vi "Build Async Parameters.vi"(8 "Error in":errorcluster, 11 "State Vars":T4 {"CompiledSettings"."Result Ch Data Refs" format="%.0x"; "CompiledSettings"."Parameter Block Data Refs"."Data Reference" format="%.0x"}) -> (0 "Error out":errorcluster, 2 "Async Parameters":T1, 3 "State Vars out":T4 {"CompiledSettings"."Result Ch Data Refs" format="%.0x"; "CompiledSettings"."Parameter Block Data Refs"."Data Reference" format="%.0x"})   [LabVIEW 2015, in "Waveform-Processing-Custom-Device Engine.lvlib"]
uses:
  Waveform-Processing-Custom-Device Engine.lvlib
  Types/Inline State Vars.ctl
  Types/Async FIFOs.ctl
  Shared/CompiledSettings.ctl
  <vilib>/NI Veristand/Custom Device API/Block Data Reference.ctl
  Built/Waveform-Processing-Custom-Device/Waveform-Processing-Custom-Device Engine Windows.llb/Data Reference.ctl
  <vilib>/NI Veristand/Custom Device API/Waveform Data Reference.ctl
  Types/Async Parameters.ctl
  <vilib>/NI VeriStand/Custom Device API/Custom Device API.lvlib
  Shared/Waveform-Processing-Custom-Device Shared.lvlib
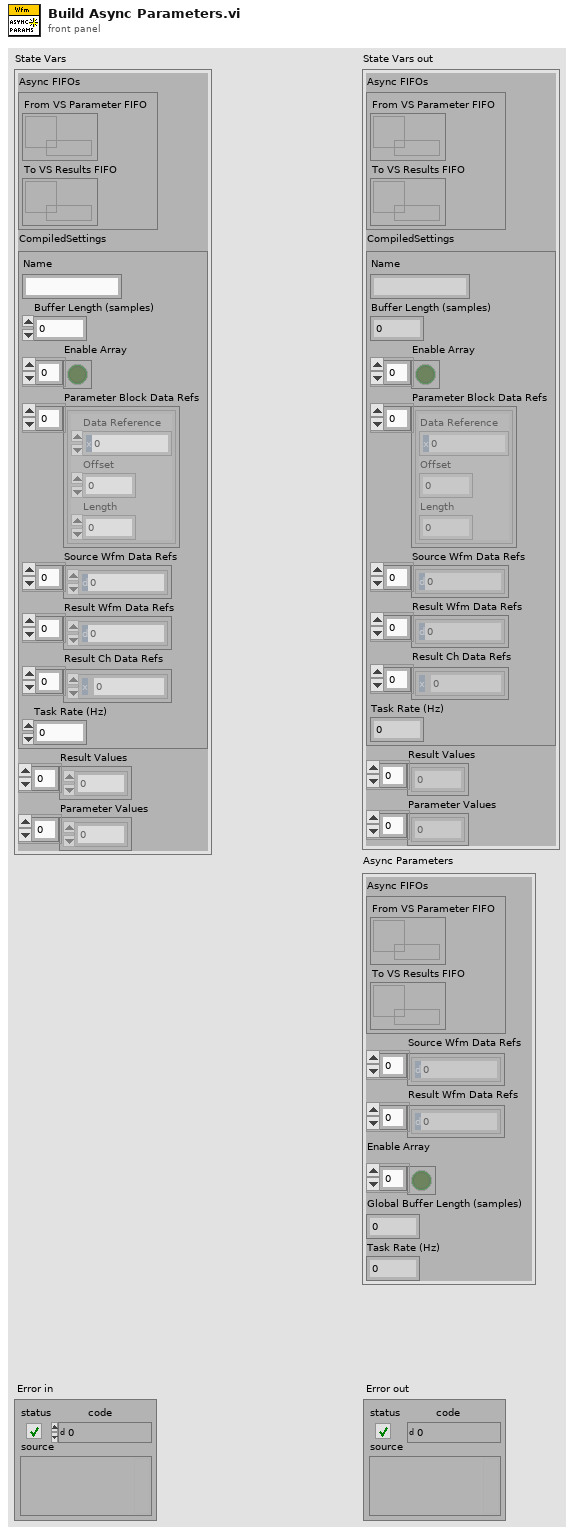
[diagram p1: front panel]
types:
  T1 = typedef "Waveform-Processing-Custom-Device Engine.lvlib/Async Parameters.ctl" = cluster{"Async FIFOs":T2, "Source Wfm Data Refs":T3[], "Result Wfm Data Refs":T3[], "Enable Array":bool[], "Global Buffer Length (samples)":dbl, "Task Rate (Hz)":dbl}
  T2 = typedef "Waveform-Processing-Custom-Device Engine.lvlib/Async FIFOs.ctl" = cluster{"From VS Parameter FIFO":refnum<k33>, "To VS Results FIFO":refnum<k33>}
  T3 = typedef "Custom Device API.lvlib/Waveform Data Reference.ctl" = i32
  T4 = typedef "Waveform-Processing-Custom-Device Engine.lvlib/Inline State Vars.ctl" = cluster{"Async FIFOs":T2, "CompiledSettings":T5, "Result Values":dbl[], "Parameter Values":dbl[]}
  T5 = typedef "Waveform-Processing-Custom-Device Shared.lvlib/CompiledSettings.ctl" = cluster{"Name":string, "Buffer Length (samples)":u32, "Enable Array":bool[], "Parameter Block Data Refs":T6[], "Source Wfm Data Refs":T3[], "Result Wfm Data Refs":T3[], "Result Ch Data Refs":T7[], "Task Rate (Hz)":dbl}
  T6 = typedef "Custom Device API.lvlib/Block Data Reference.ctl" = cluster{"Data Reference":T7, "Offset":u64, "Length":u64}
  T7 = typedef "Custom Device API.lvlib/Data Reference.ctl" = i32
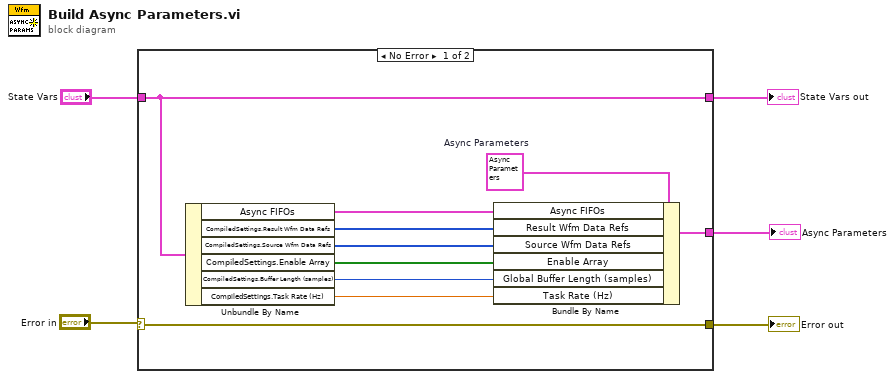
[diagram p0: block diagram]
diagram:
  n1 = case shown="No Error" "Error in" {
    selector: "Error in" -> [w11 w17]
    tunnel: [w11 w17] -> w4
    tunnel: "State Vars" -> [w12 w16]
    tunnel: [w12 w16] -> w2
    tunnel: [w13 _] -> w1
    frame No Error {
      w15 = T1 {"Async FIFOs"={"From VS Parameter FIFO"=refnum, "To VS Results FIFO"=refnum}, "Source Wfm Data Refs"=[], "Result Wfm Data Refs"=[], "Enable Array"=[], "Global Buffer Length (samples)"=0.0, "Task Rate (Hz)"=0.0}  # Async Parameters
      n2 = Unbundle By Name(w12) -> ("Async FIFOs"=w14:T2, "CompiledSettings.Result Wfm Data Refs"=w10:T3[], "CompiledSettings.Source Wfm Data Refs"=w9:T3[], "CompiledSettings.Enable Array"=w8:bool[], "CompiledSettings.Buffer Length (samples)"=w7:u32, "CompiledSettings.Task Rate (Hz)"=w6:dbl)
      n3 = Bundle By Name(cluster=w15, "Async FIFOs"=w14, "Result Wfm Data Refs"=w10, "Source Wfm Data Refs"=w9, "Enable Array"=w8, "Global Buffer Length (samples)"=w7, "Task Rate (Hz)"=w6) -> (w13:T1)
    }
    frame Error {
    }
  }
  "Error out" <- w4
  "State Vars out" <- w2
  "Async Parameters" <- w1
